vi "overlay_particle(subVI).vi"(8 "error in (no error)":errorcluster, 10 "image source":T1, 11 "image dst":T1) -> (0 "error out":errorcluster, 1 "Particle Reports (Real-World)":T2(array[cluster]) {"Orientation" format="%.2f"; "Dimensions"."Height" format="%.2f"; "Dimensions"."Width" format="%.2f"; "Center of Mass"."Y" format="%.2f"; "Center of Mass"."X" format="%.2f"; "Bounding Rect"."Bottom" format="%.2f"; "Bounding Rect"."Right" format="%.2f"; "Bounding Rect"."Top" format="%.2f"; "Bounding Rect"."Left" format="%.2f"; "Number of Holes" format="%.2f"; "Area" format="%.2f"}, 2 "Particle Reports (Pixels)":T2(array[cluster]) {"Orientation" format="%.2f"; "Dimensions"."Height" format="%.2f"; "Dimensions"."Width" format="%.2f"; "Center of Mass"."Y" format="%.2f"; "Center of Mass"."X" format="%.2f"; "Bounding Rect"."Bottom" format="%.2f"; "Bounding Rect"."Right" format="%.2f"; "Bounding Rect"."Top" format="%.2f"; "Bounding Rect"."Left" format="%.2f"; "Number of Holes" format="%.2f"; "Area" format="%.2f"}, 3 "image Out":T1, 5 "number of particle":i32)   [LabVIEW 2020]
uses:
  <vilib>/vision/Image Controls.llb/IMAQ Image.ctl
  <vilib>/vision/NI_Vision_Development_Module.lvlib
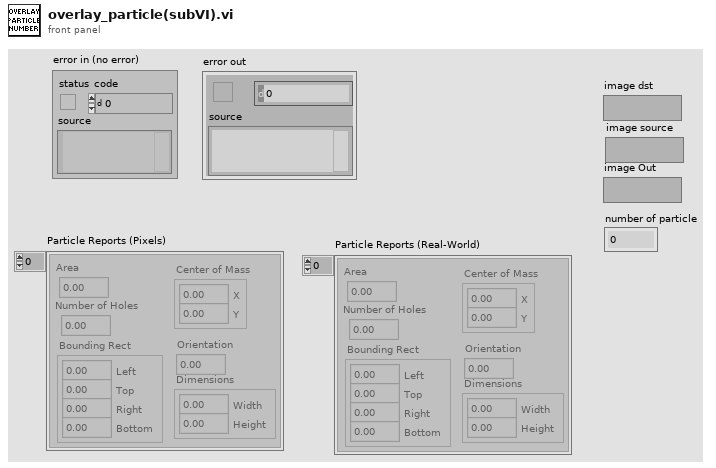
[diagram p1: front panel]
types:
  T1 = typedef "IMAQ Image.ctl" = refnum<image>
  T2 = cluster{"Area":dbl, "Number of Holes":dbl, "Bounding Rect":cluster{"Left":dbl, "Top":dbl, "Right":dbl, "Bottom":dbl}, "Center of Mass":cluster{"X":dbl, "Y":dbl}, "Orientation":dbl, "Dimensions":cluster{"Width":dbl, "Height":dbl}}[]
  T3 = cluster{"Desired Font (Application)":enum16{"User-specified Font", "Application Font", "System Font", "Dialog Font"}, "[User-specified Font]":cluster{"Font Name":string, "Size":i16, "Strikeout?":bool, "Italic?":bool, "Underline?":bool, "Outline?":bool, "Shadow?":bool, "Bold?":bool, "Rotation Angle":dbl}, "Horizontal Alignment":i16, "Vertical Alignment":i16}
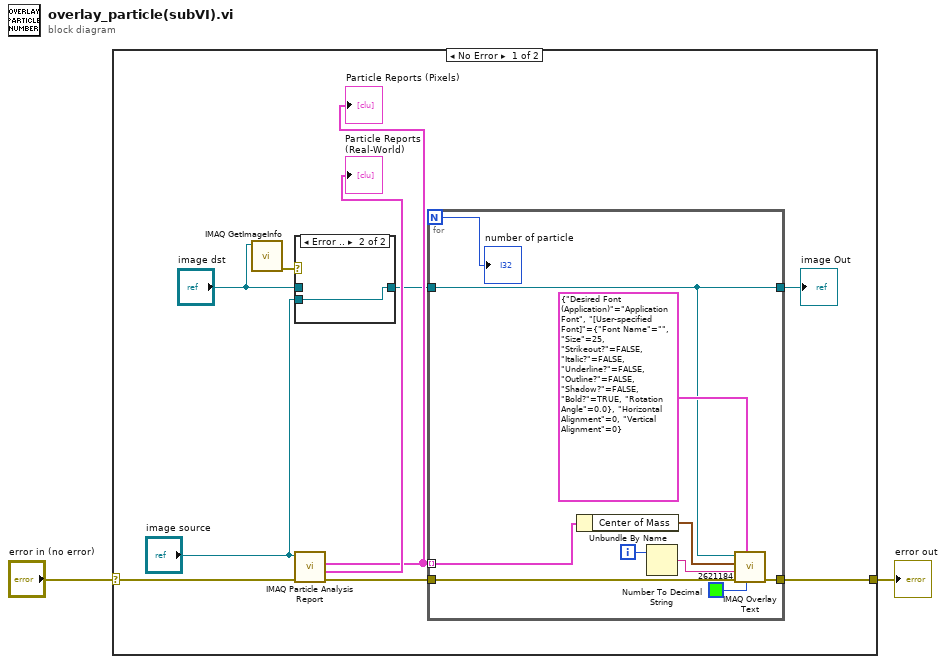
[diagram p0: block diagram]
diagram:
  n1 = case shown="No Error" "error in (no error)" {
    selector: "error in (no error)" -> [w11 w25]
    tunnel: [w10 w25] -> w2
    frame No Error {
      n2 = call "IMAQ GetImageInfo"("Image"="image dst") -> ("error out"=w7:errorcluster)  [unwired: 3 in, 7 out]
      n3 = case shown="Error .." w7 {
        tunnel: [w13 w14] -> w6
        tunnel: "image dst" -> [w13 _]
        tunnel: "image source" -> [_ w14]
        frame No Error {
        }
        frame Error {
        }
      }
      n4 = call "IMAQ Particle Analysis Report"("error in (no error)"=w11, "Image"="image source") -> ("error out"=w9:errorcluster, "Particle Reports (Real-World)"=→"Particle Reports (Real-World)":T2, "Particle Reports (Pixels)"=w8:T2)  [unwired: 4 in, 3 out]
      "Particle Reports (Pixels)" <- w8
      n5 = for {
        N -> [w16]
        tunnel: [w19] -> w10
        tunnel: w8 -> [w18] mode=indexing
        tunnel: w9 -> [w17]
        tunnel: w6 -> [w15]
        tunnel: [w15] -> w4
        i -> [w23]
        n6 = Unbundle By Name(w18) -> ("Center of Mass"=w24:cluster{"X":dbl, "Y":dbl})
        n7 = Number To Decimal String(number=w23) -> (decimal integer string=w22:string)  [unwired: 1 in]
        n8 = call "IMAQ Overlay Text"("Text Color (black)"=u32 2621184, "Font, Size & Style"=T3 {"Desired Font (Application)"=enum."Application Font", "[User-specified Font]"={"Font Name"="", "Size"=25, "Strikeout?"=FALSE, "Italic?"=FALSE, "Underline?"=FALSE, "Outline?"=FALSE, "Shadow?"=FALSE, "Bold?"=TRUE, "Rotation Angle"=0.0}, "Horizontal Alignment"=0, "Vertical Alignment"=0}, "error in (no error)"=w17, "String"=w22, "Origin"=w24, "Image"=w15) -> ("error out"=w19:errorcluster)  [unwired: 4 in, 1 out]
        "number of particle" <- w16
      }
      "image Out" <- w4
    }
    frame Error {
    }
  }
  "error out" <- w2
